vi "DMS_Read.vi"(8 "error in (no error)":errorcluster) -> (0 "error out":errorcluster, 1 "DMS":T1)   [LabVIEW 2020]
uses:
  Controls/DMS_Control.ctl
  Controls/dms_BOOL.ctl
panel:
  in  "NO PLAN":bool
  in  "CHANGE OVER":bool
  in  "NO MATERIAL":bool
  in  "BREAK DOWN":bool
  in  "LINE RUNNING":bool
  in  "DMS 2":T1
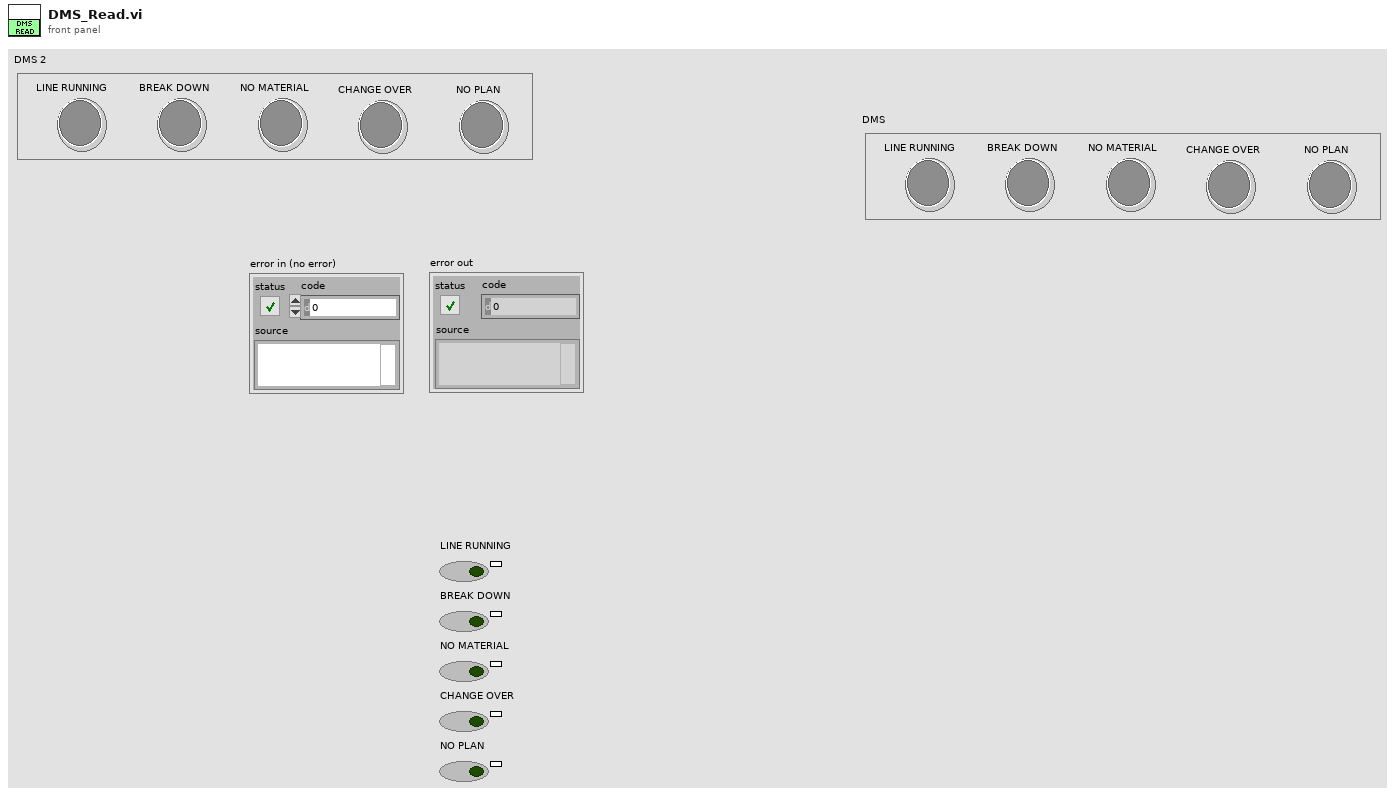
[diagram p1: front panel]
types:
  T1 = typedef "DMS_Control.ctl" = cluster{"LINE RUNNING":T2, "BREAK DOWN":T2, "NO MATERIAL":T2, "CHANGE OVER":T2, "NO PLAN":T2}
  T2 = typedef "dms_BOOL.ctl" = bool
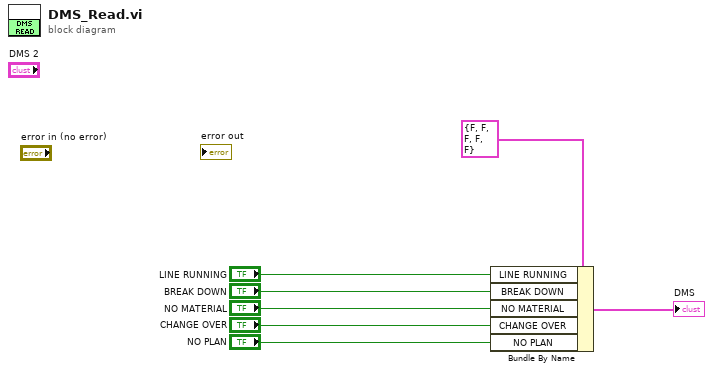
[diagram p0: block diagram]
diagram:
  n1 = Bundle By Name(cluster=T1 {"LINE RUNNING"=FALSE, "BREAK DOWN"=FALSE, "NO MATERIAL"=FALSE, "CHANGE OVER"=FALSE, "NO PLAN"=FALSE} ("DMS"), "LINE RUNNING"="LINE RUNNING", "BREAK DOWN"="BREAK DOWN", "NO MATERIAL"="NO MATERIAL", "CHANGE OVER"="CHANGE OVER", "NO PLAN"="NO PLAN") -> (→"DMS":T1)
